vi "SimpleJsonNQuery.vi"(8 "error in":errorcluster, 10 "Lookups":string[](array[string]), 11 "JsonString":string) -> (0 "error out":errorcluster, 2 "Value As Numeric":dbl[](array[numeric]), 3 "Values As String":string[](array[string]))   [LabVIEW 2020]
doc: "Given a json string, extract values at the specified lookup strings ('keys')"
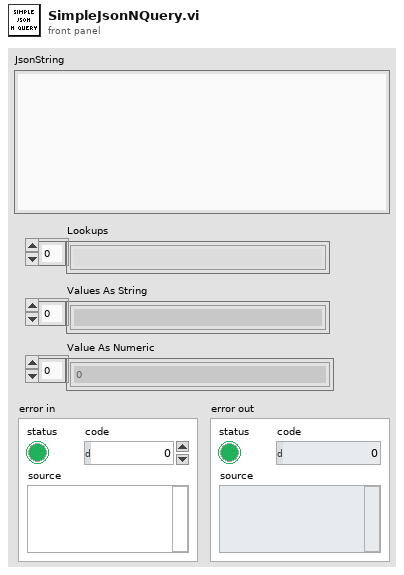
[diagram p1: front panel]
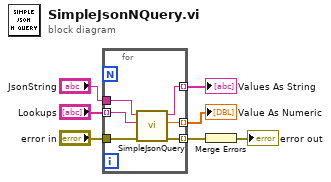
[diagram p0: block diagram]
diagram:
  n1 = for {
    tunnel: "JsonString" -> [w13]
    tunnel: "Lookups" -> [w12] mode=indexing
    tunnel: [w11] -> w5 mode=indexing
    tunnel: [w10] -> w4 mode=indexing
    tunnel: "error in" -> [w9]
    tunnel: [w8] -> w2 mode=indexing
    n2 = call "SimpleJsonQuery.vi"("error in"=w9, "Lookup"=w12, "JsonString"=w13) -> ("error out"=w8:errorcluster, "Value As Numeric"=w11:dbl, "Value As String"=w10:string)  [unwired: 6 in]
  }
  "Values As String" <- w4
  "Value As Numeric" <- w5
  n3 = Merge Errors(w2) -> (→"error out":errorcluster)
